vi "xiC - TwoButtonDialog.vi"(6 "Icon":i32(ring)=32 items=["None"=0, "Hand, Error, Stop"=16, "Question"=32, "Exclamation, Warning"=48, "Asterisk, Information"=64], 7 "Caption":string="xiControl", 8 "error in (no error)":errorcluster, 9 "Button":i32(ring)=4 items=["OK", "OKCancel", "AbortRetryIgnore", "YesNoCancel", "YesNo", "RetryCancel"], 11 "Text":string="This is Dialog") -> (0 "error out":errorcluster, 3 "Show":i32(ring) items=["None", "OK", "Cancel", "Abort", "Retry", "Ignore", "Yes", "No"])   [LabVIEW 2013]
uses:
  System.Windows.Forms
panel:
  in  "defaultButton":i32(ring) items=["Button1"=0, "Button2"=256, "Button3"=512]
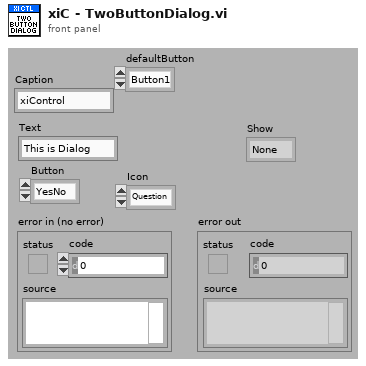
[diagram p1: front panel]
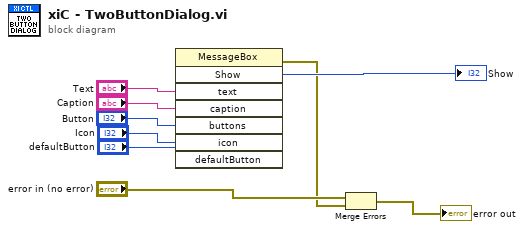
[diagram p0: block diagram]
diagram:
  n1 = invoke class="MessageBox" method="Show"("text"="Text", "caption"="Caption", "buttons"="Button", "icon"="Icon", "defaultButton"="defaultButton") -> (error out=w6:errorcluster, "Show"=→"Show":i32)  [unwired: 3 in, 6 out]
  n2 = Merge Errors("error in (no error)", w6) -> (→"error out":errorcluster)
